vi "Run.vi"(8 "error in (no error)":errorcluster caption="entrée d'erreur (pas d'erreur)", 11 "Sparse_Uncorrelated.lvclass":refnum<class "Sparse_Uncorrelated.lvclass">) -> (0 "error out":errorcluster caption="sortie d'erreur", 2 "Data":T1, 3 "Sparse_Uncorrelated.lvclass":refnum<class "Sparse_Uncorrelated.lvclass">)   [LabVIEW 2020, in "Sparse_Uncorrelated.lvclass"]
doc: "Returns :\n\nX : array of shape [n_samples, n_features]\nThe input samples.\n\ny : array of shape [n_samples]\nThe output values."
uses:
  Sparse_Uncorrelated.lvclass
  Sparse_Uncorrelated.lvclass/Sparse_Uncorrelated.ctl
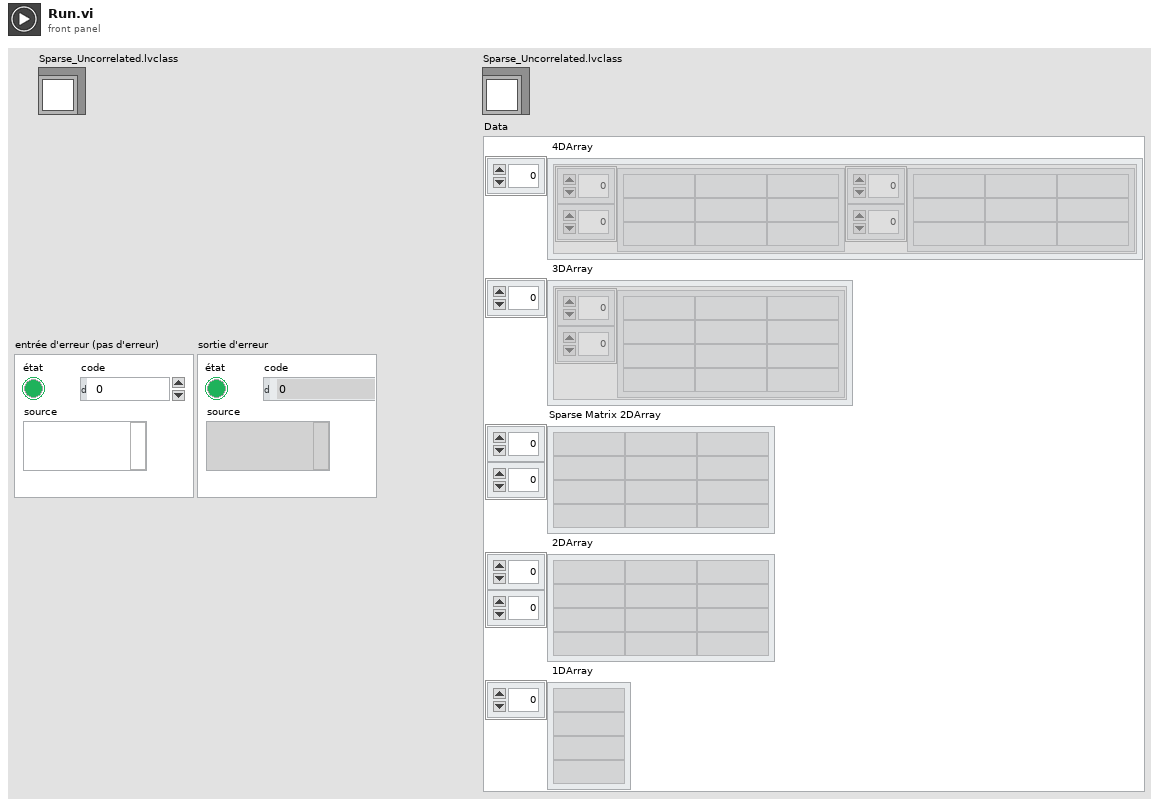
[diagram p1: front panel]
types:
  T1 = cluster{" 4DArray":cluster{"1":string[][], "2":string[][]}[], " 3DArray":cluster{"Tableau":string[][]}[], "Sparse Matrix 2DArray":string[][], " 2DArray":string[][], " 1DArray":string[]}
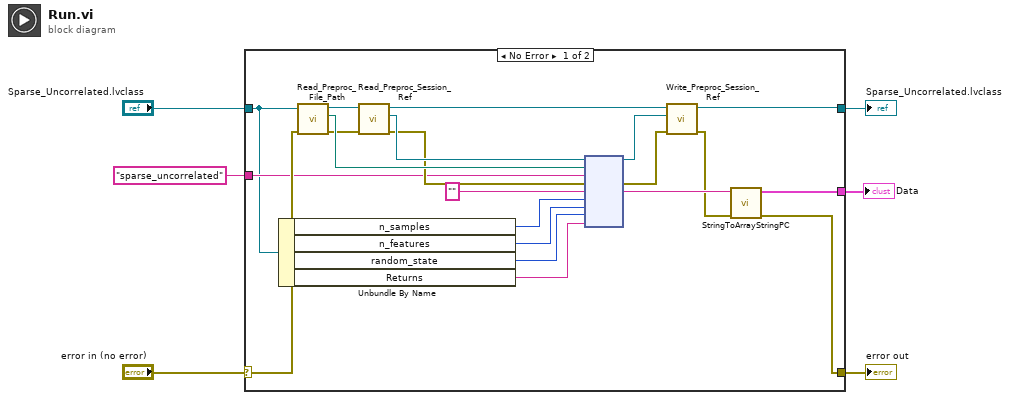
[diagram p0: block diagram]
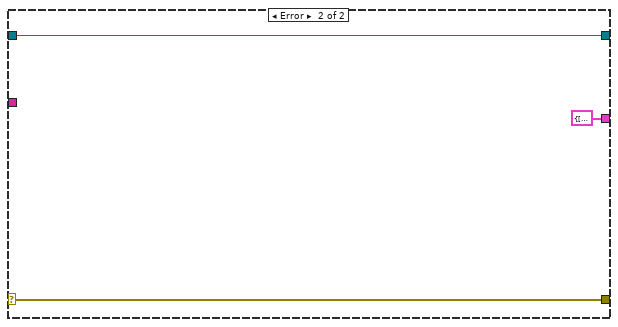
[diagram p2: hidden frame]
diagram:
  n1 = case shown="No Error" "error in (no error)" {
    selector: "error in (no error)" -> [w19 w30]
    tunnel: [w8 w30] -> w5
    tunnel: [w11 w29] -> w3
    tunnel: "Sparse_Uncorrelated.lvclass" -> [w17 w29]
    tunnel: "sparse_uncorrelated" -> [w18 _]
    tunnel: [w7 T1 {" 4DArray"=[], " 3DArray"=[], "Sparse Matrix 2DArray"=[], " 2DArray"=[], " 1DArray"=[]} ("Data")] -> w1
    frame No Error {
      n2 = Unbundle By Name(w17) -> ("n_samples"=w16:u32, "n_features"=w15:i32, "random_state"=w14:i32, "Returns"=w13:string)
      n3 = call-dynamic "Read_Preproc_File_Path.vi"("error in (no error)"=w19, "Python in"=w17) -> ("error out"=w22:errorcluster, "File_Path"=w25:path, "Python out"=w27:refnum<class "Sparse_Uncorrelated.lvclass">)  [unwired: 7 in]
      n4 = call-dynamic "Read_Preproc_Session_Ref.vi"("error in (no error)"=w22, "Python in"=w27) -> ("error out"=w23:errorcluster, "Session_ref"=w24:refnum<k35>, "Python out"=w26:refnum<class "Sparse_Uncorrelated.lvclass">)  [unwired: 7 in]
      n5 = node(w24, w25, w18, w23, "", w16, w15, w14, w13) -> (w20:refnum<k35>, w12:errorcluster, w10:string)  [unwired: 4 in, 2 out]
      n6 = call-dynamic "Write_Preproc_Session_Ref.vi"("error in (no error)"=w12, "Session_ref"=w20, "Python in"=w26) -> ("error out"=w9:errorcluster, "Python out"=w11:refnum<class "Sparse_Uncorrelated.lvclass">)  [unwired: 7 in]
      n7 = call "StringToArrayStringPC.vi"("sortie d'erreur"=w9, "Return value"=w10) -> ("sortie d'erreur"=w8:errorcluster, "Data"=w7:T1)  [unwired: 8 in]
    }
    frame Error {
    }
  }
  "error out" <- w5
  "Sparse_Uncorrelated.lvclass" <- w3
  "Data" <- w1
